vi "MoveScanFunc.vi"(6 "Multi ScanPar":bool[](array[boolean]), 7 "ActScanPar":bool[](array[boolean]), 8 "ErrorIn(No Error)":errorcluster caption="entrée d'erreur (pas d'erreur)", 9 "ScanFuncIn":string[][](array[string]), 10 "Dir(Up:T)":bool, 11 "Value":string) -> (0 "sortie d'erreur":errorcluster, 1 "ScanFuncOut":string[][](array[string]), 4 "Multi ScanParOut":bool[](array[boolean]), 5 "ActScanParOut":bool[](array[boolean]))   [LabVIEW 2019]
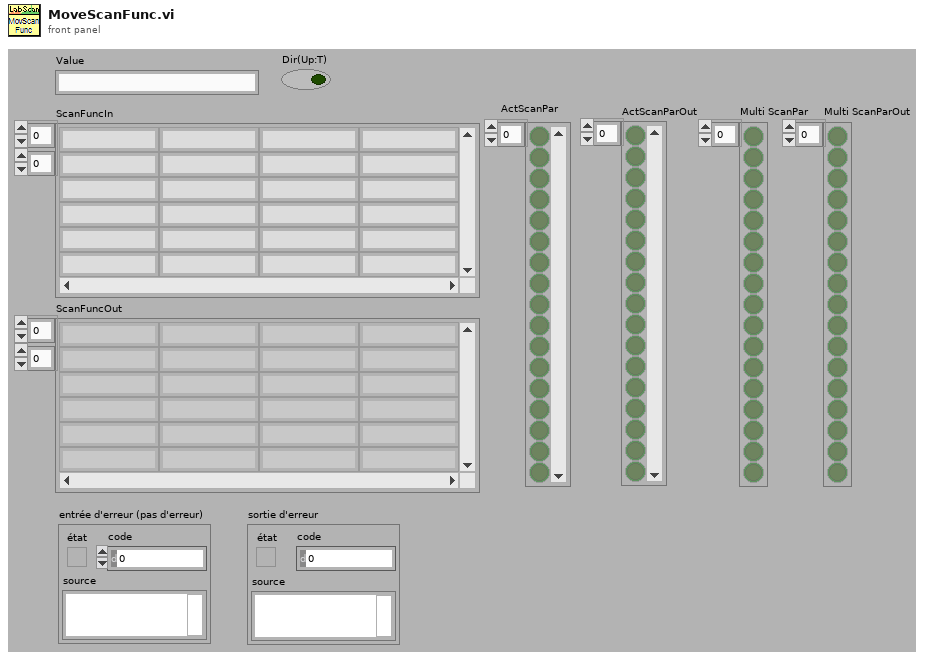
[diagram p1: front panel]
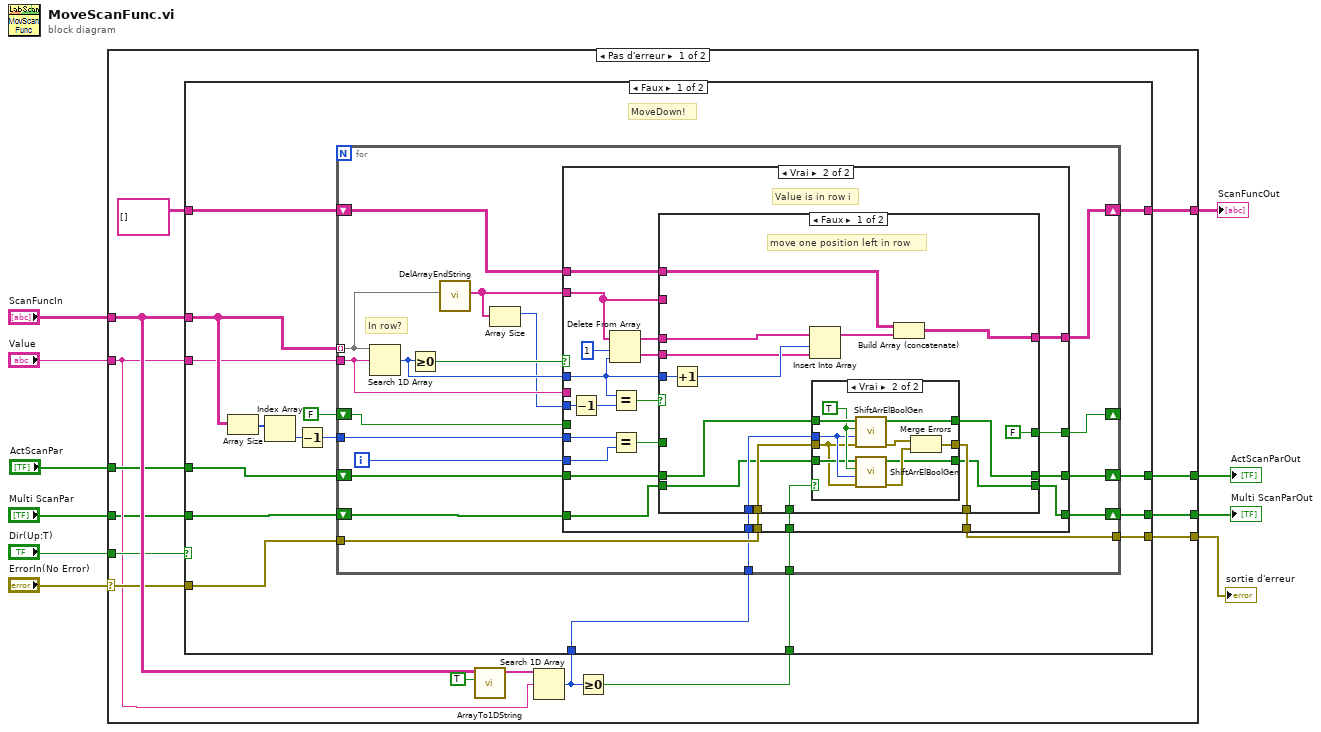
[diagram p0: block diagram]
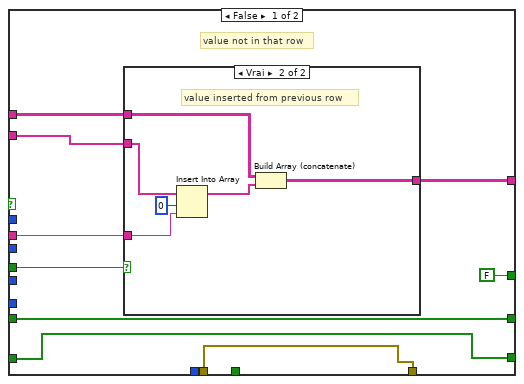
[diagram p2: hidden frame]
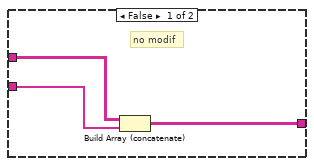
[diagram p3: hidden frame]
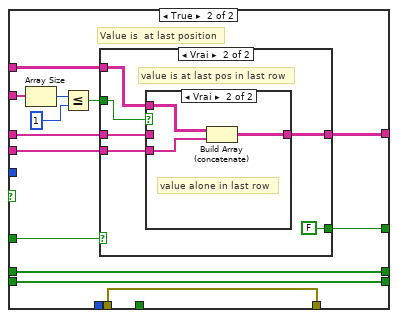
[diagram p5: hidden frame]
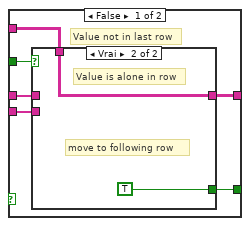
[diagram p6: hidden frame]
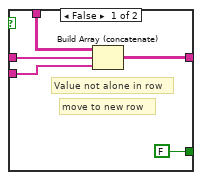
[diagram p7: hidden frame]
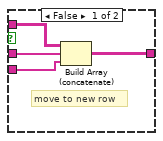
[diagram p8: hidden frame]
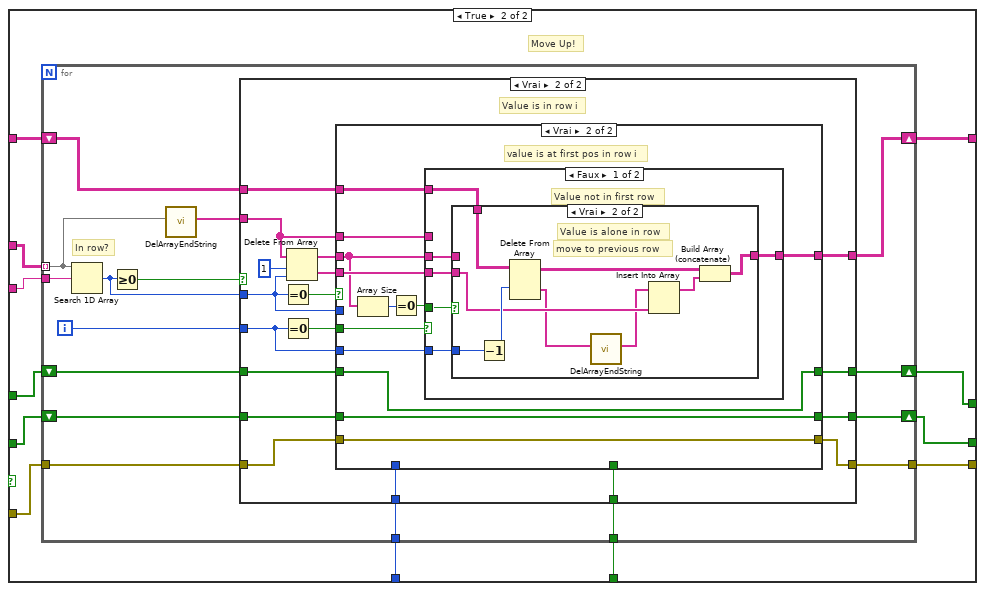
[diagram p9: hidden frame]
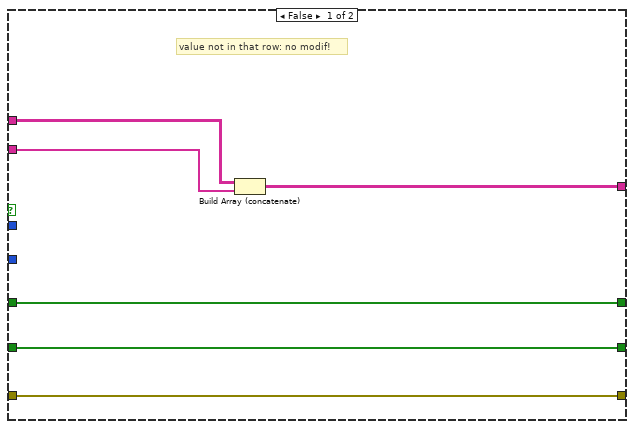
[diagram p10: hidden frame]
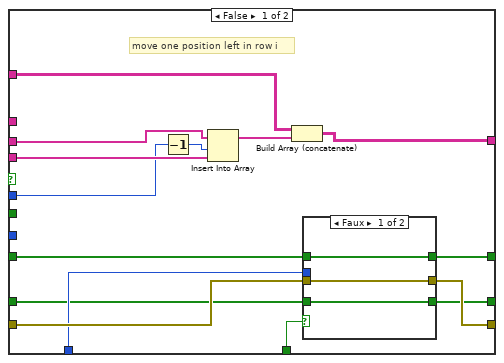
[diagram p11: hidden frame]
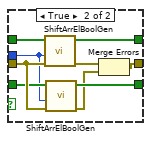
[diagram p12: hidden frame]
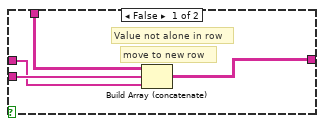
[diagram p13: hidden frame]
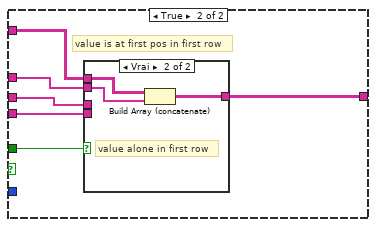
[diagram p14: hidden frame]
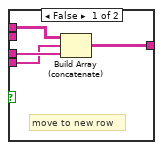
[diagram p15: hidden frame]
diagram:
  n1 = case shown="Pas d'erreur" "ErrorIn(No Error)" {
    selector: "ErrorIn(No Error)" -> [w20 w296]
    tunnel: "Value" -> [w13 _]
    tunnel: "ScanFuncIn" -> [w24 w295]
    tunnel: "Dir(Up:T)" -> [w21 _]
    tunnel: [w19 w296] -> w6
    tunnel: [w23 w295] -> w5
    tunnel: "ActScanPar" -> [w22 w294]
    tunnel: [w18 w294] -> w3
    tunnel: "Multi ScanPar" -> [w12 w293]
    tunnel: [w11 w293] -> w1
    frame No Error {
      n2 = call <userlib>:"ArrayTo1DString.vi"("DelArrEnd(F)"=TRUE ("DelArrEnd"), "tableau"=w24) -> ("Array Out"=w17:string[])  [unwired: 7 in, 2 out]
      n3 = Search 1D Array(1D array=w17, element=w13) -> (index of element=w14:i32)  [unwired: 1 in]
      n4 = Greater Or Equal To 0?(x=w14) -> (x >= 0?=w15:bool)
      n5 = case shown="Faux" w21 {
        tunnel: w13 -> [w31 w179]
        tunnel: string[][] [] -> [w41 w181]
        tunnel: [w40 w178] -> w23
        tunnel: w24 -> [w32 w180]
        tunnel: w22 -> [w28 w175]
        tunnel: w20 -> [w35 w176]
        tunnel: [w34 w177] -> w19
        tunnel: [w33 w173] -> w18
        tunnel: w15 -> [w30 w172]
        tunnel: w14 -> [w29 w174]
        tunnel: w12 -> [w27 w171]
        tunnel: [w26 w170] -> w11
        frame False {
          # "MoveDown!"
          n6 = Array Size(array=w32) -> (size(s)=w39:i32[])
          n7 = Index Array(array=w39) -> (element=w38:i32)  [unwired: 1 in]
          n8 = Decrement(x=w38) -> (x-1=w37:i32)
          n9 = for {
            tunnel: w32 -> [w52] mode=indexing
            tunnel: w31 -> [w53]
            shift-right: [w58] -> w40
            shift-left: w41 -> [w57]
            tunnel: w37 -> [w56]
            shift-right: [w55] -> _
            shift-left: FALSE -> [w54]
            tunnel: w35 -> [w49]
            tunnel: [w48] -> w34
            tunnel: w30 -> [w46]
            tunnel: w29 -> [w45]
            shift-right: [w47] -> w33
            shift-left: w28 -> [w44]
            shift-right: [w43] -> w26
            shift-left: w27 -> [w42]
            i -> [w59]
            # "In row?"
            n10 = Search 1D Array(1D array=w52, element=w53) -> (index of element=w60:i32)  [unwired: 1 in]
            n11 = Greater Or Equal To 0?(x=w60) -> (x >= 0?=w61:bool)
            n12 = call <userlib>:"DelArrayEndString.vi"("Array In"=w52) -> ("Array Out"=w50:string[])  [unwired: 9 in, 1 out]
            n13 = Array Size(array=w50) -> (size(s)=w51:i32)
            n14 = case shown="Vrai" w61 {
              tunnel: w60 -> [_ w88]
              tunnel: w50 -> [w68 w97]
              tunnel: [w69 w98] -> w58
              tunnel: w59 -> [_ w91]
              tunnel: w57 -> [w70 w96]
              tunnel: w51 -> [_ w95]
              tunnel: w56 -> [_ w92]
              tunnel: [FALSE w90] -> w55
              tunnel: w54 -> [w66 _]
              tunnel: w53 -> [w65 _]
              tunnel: w46 -> [_ w87]
              tunnel: w44 -> [w63 w82]
              tunnel: w49 -> [w64 w86]
              tunnel: w45 -> [_ w85]
              tunnel: [w64 w84] -> w48
              tunnel: [w63 w83] -> w47
              tunnel: [w62 w81] -> w43
              tunnel: w42 -> [w62 w80]
              frame False {
                # "value not in that row"
                n15 = case shown="Vrai" w66 {
                  tunnel: w70 -> [w73 w77]
                  tunnel: [w72 w75] -> w69
                  tunnel: w68 -> [w71 w79]
                  tunnel: w65 -> [_ w78]
                  frame False {
                    # "no modif"
                    n16 = Build Array (concatenate)(w73, w71) -> (w72:string[][])
                  }
                  frame True {
                    # "value inserted from previous row"
                    n17 = Insert Into Array(array=w79, index=0 ("indice"), new element=w78) -> (w76:string[])
                    n18 = Build Array (concatenate)(w77, w76) -> (w75:string[][])
                  }
                }
              }
              frame True {
                # "Value is in row i"
                n19 = Decrement(x=w95) -> (x-1=w89:i32)
                n20 = Delete From Array(array=w97, length=1 ("longueur"), index=w88) -> (deleted portion=w99:string[], array with subset deleted=w100:string[])
                n21 = Equal?(x=w88, y=w89) -> (x = y?=w94:bool)
                n22 = Equal?(x=w92, y=w91) -> (x = y?=w93:bool)
                n23 = case shown="Faux" w94 {
                  tunnel: w100 -> [w110 w139]
                  tunnel: w99 -> [w116 w142]
                  tunnel: w88 -> [w115 _]
                  tunnel: [w114 w141] -> w98
                  tunnel: w93 -> [_ w143]
                  tunnel: w97 -> [_ w137]
                  tunnel: w96 -> [w112 w140]
                  tunnel: [FALSE w134] -> w90
                  tunnel: w87 -> [w109 _]
                  tunnel: w82 -> [w104 w132]
                  tunnel: w86 -> [w108 w133]
                  tunnel: w85 -> [w107 _]
                  tunnel: [w106 w133] -> w84
                  tunnel: [w105 w132] -> w83
                  tunnel: [w102 w131] -> w81
                  tunnel: w80 -> [w103 w131]
                  frame False {
                    # "move one position left in row"
                    n24 = Increment(x=w115) -> (x+1=w117:i32)
                    n25 = Insert Into Array(array=w110, index=w117, new element=w116) -> (w113:string[])
                    n26 = case shown="Vrai" w109 {
                      tunnel: w104 -> [w120 w130]
                      tunnel: w108 -> [w119 w123]
                      tunnel: w107 -> [_ w127]
                      tunnel: [w119 w122] -> w106
                      tunnel: [w120 w129] -> w105
                      tunnel: w103 -> [w118 w124]
                      tunnel: [w118 w125] -> w102
                      frame False {
                      }
                      frame True {
                        w128 = TRUE ("Dir(DownFalse)")
                        n27 = call <userlib>:"ShiftArrElBoolGen.vi"("ErrorIn(No Error)"=w123, "Index"=w127, "Dir(DownFalse)"=w128, "Array In"=w130) -> ("sortie d'erreur"=w121:errorcluster, "Array Out"=w129:bool[])  [unwired: 5 in, 1 out]
                        n28 = call <userlib>:"ShiftArrElBoolGen.vi"("ErrorIn(No Error)"=w123, "Index"=w127, "Dir(DownFalse)"=w128, "Array In"=w124) -> ("sortie d'erreur"=w126:errorcluster, "Array Out"=w125:bool[])  [unwired: 5 in, 1 out]
                        n29 = Merge Errors(w121, w126) -> (w122:errorcluster)
                      }
                    }
                    n30 = Build Array (concatenate)(w112, w113) -> (w114:string[][])
                  }
                  frame True {
                    # "Value is  at last position"
                    n31 = Array Size(array=w137) -> (size(s)=w136:i32)
                    n32 = Less Or Equal?(x=w136, y=1) -> (x <= y?=w138:bool)
                    n33 = case shown="Vrai" w143 {
                      tunnel: w139 -> [w146 w158]
                      tunnel: w142 -> [w149 w159]
                      tunnel: [w148 w162] -> w141
                      tunnel: w140 -> [w147 w161]
                      tunnel: w138 -> [w145 w160]
                      tunnel: [w144 FALSE] -> w134
                      frame False {
                        # "Value not in last row"
                        n34 = case shown="Vrai" w145 {
                          tunnel: w149 -> [w152 _]
                          tunnel: [w154 w156] -> w148
                          tunnel: w147 -> [w153 w156]
                          tunnel: w146 -> [w151 _]
                          tunnel: [FALSE TRUE] -> w144
                          frame False {
                            # "Value not alone in row"
                            # "move to new row"
                            n35 = Build Array (concatenate)(w153, w151, w152) -> (w154:string[][])
                          }
                          frame True {
                            # "Value is alone in row"
                            # "move to following row"
                          }
                        }
                      }
                      frame True {
                        # "value is at last pos in last row"
                        n36 = case shown="Vrai" w160 {
                          tunnel: [w165 w169] -> w162
                          tunnel: w161 -> [w166 w168]
                          tunnel: w159 -> [w164 w167]
                          tunnel: w158 -> [w163 _]
                          frame False {
                            # "move to new row"
                            n37 = Build Array (concatenate)(w166, w163, w164) -> (w165:string[][])
                          }
                          frame True {
                            # "value alone in last row"
                            n38 = Build Array (concatenate)(w168, w167) -> (w169:string[][])
                          }
                        }
                      }
                    }
                  }
                }
              }
            }
          }
        }
        frame True {
          # "Move Up!"
          n39 = for {
            tunnel: w180 -> [w191] mode=indexing
            tunnel: w179 -> [w197]
            shift-right: [w193] -> w178
            shift-left: w181 -> [w192]
            tunnel: [w189] -> w177
            tunnel: w176 -> [w188]
            tunnel: w174 -> [w186]
            shift-right: [w185] -> w173
            shift-left: w175 -> [w187]
            tunnel: w172 -> [w184]
            shift-right: [w182] -> w170
            shift-left: w171 -> [w183]
            i -> [w194]
            # "In row?"
            n40 = Search 1D Array(1D array=w191, element=w197) -> (index of element=w195:i32)  [unwired: 1 in]
            n41 = Greater Or Equal To 0?(x=w195) -> (x >= 0?=w196:bool)
            n42 = call <userlib>:"DelArrayEndString.vi"("Array In"=w191) -> ("Array Out"=w190:string[])  [unwired: 9 in, 1 out]
            n43 = case shown="Vrai" w196 {
              tunnel: w195 -> [_ w217]
              tunnel: w190 -> [w201 w214]
              tunnel: [w202 w216] -> w193
              tunnel: w194 -> [_ w212]
              tunnel: w192 -> [w203 w213]
              tunnel: [w200 w210] -> w189
              tunnel: w188 -> [w200 w211]
              tunnel: [w199 w209] -> w185
              tunnel: w187 -> [w199 w208]
              tunnel: w186 -> [_ w207]
              tunnel: w184 -> [_ w206]
              tunnel: w183 -> [w198 w205]
              tunnel: [w198 w204] -> w182
              frame False {
                # "value not in that row: no modif!"
                n44 = Build Array (concatenate)(w203, w201) -> (w202:string[][])
              }
              frame True {
                # "Value is in row i"
                n45 = Equal To 0?(x=w217) -> (x = 0?=w220:bool)
                n46 = Equal To 0?(x=w212) -> (x = 0?=w215:bool)
                n47 = Delete From Array(array=w214, length=1 ("longueur"), index=w217) -> (deleted portion=w218:string[], array with subset deleted=w219:string[])
                n48 = case shown="Vrai" w220 {
                  tunnel: w219 -> [w233 w254]
                  tunnel: w218 -> [w235 w259]
                  tunnel: w217 -> [w234 _]
                  tunnel: [w232 w258] -> w216
                  tunnel: w215 -> [_ w260]
                  tunnel: w214 -> [_ w257]
                  tunnel: w213 -> [w230 w256]
                  tunnel: w212 -> [_ w255]
                  tunnel: w211 -> [w229 w251]
                  tunnel: [w228 w251] -> w210
                  tunnel: [w227 w250] -> w209
                  tunnel: w208 -> [w226 w250]
                  tunnel: w207 -> [w225 _]
                  tunnel: w206 -> [w224 _]
                  tunnel: w205 -> [w223 w249]
                  tunnel: [w222 w249] -> w204
                  frame False {
                    # "move one position left in row i"
                    n49 = Decrement(x=w234) -> (x-1=w236:i32)
                    n50 = Insert Into Array(array=w233, index=w236, new element=w235) -> (w231:string[])
                    n51 = Build Array (concatenate)(w230, w231) -> (w232:string[][])
                    n52 = case shown="Faux" w224 {
                      tunnel: w226 -> [w239 w248]
                      tunnel: w229 -> [w238 w245]
                      tunnel: w225 -> [_ w240]
                      tunnel: [w238 w243] -> w228
                      tunnel: [w239 w246] -> w227
                      tunnel: w223 -> [w237 w241]
                      tunnel: [w237 w244] -> w222
                      frame False {
                      }
                      frame True {
                        n53 = call <userlib>:"ShiftArrElBoolGen.vi"("ErrorIn(No Error)"=w245, "Index"=w240, "Array In"=w248) -> ("sortie d'erreur"=w247:errorcluster, "Array Out"=w246:bool[])  [unwired: 6 in, 1 out]
                        n54 = call <userlib>:"ShiftArrElBoolGen.vi"("ErrorIn(No Error)"=w245, "Index"=w240, "Array In"=w241) -> ("sortie d'erreur"=w242:errorcluster, "Array Out"=w244:bool[])  [unwired: 6 in, 1 out]
                        n55 = Merge Errors(w247, w242) -> (w243:errorcluster)
                      }
                    }
                  }
                  frame True {
                    # "value is at first pos in row i"
                    n56 = Array Size(array=w254) -> (size(s)=w253:i32)
                    n57 = Equal To 0?(x=w253) -> (x = 0?=w252:bool)
                    n58 = case shown="Faux" w260 {
                      tunnel: w254 -> [w263 w280]
                      tunnel: w259 -> [w266 w281]
                      tunnel: [w265 w285] -> w258
                      tunnel: w257 -> [_ w283]
                      tunnel: w256 -> [w264 w284]
                      tunnel: w255 -> [w262 _]
                      tunnel: w252 -> [w261 w282]
                      frame False {
                        # "Value not in first row"
                        n59 = case shown="Vrai" w261 {
                          tunnel: w266 -> [w270 w274]
                          tunnel: [w269 w271] -> w265
                          tunnel: w264 -> [w268 w278]
                          tunnel: w263 -> [w267 _]
                          tunnel: w262 -> [_ w279]
                          frame False {
                            # "Value not alone in row"
                            # "move to new row"
                            n60 = Build Array (concatenate)(w268, w270, w267) -> (w269:string[][])
                          }
                          frame True {
                            # "Value is alone in row"
                            # "move to previous row"
                            n61 = Decrement(x=w279) -> (x-1=w275:i32)
                            n62 = Delete From Array(array=w278, index (row)=w275) -> (deleted portion=w273:string[], array with subset deleted=w277:string[][])  [unwired: 2 in]
                            n63 = call <userlib>:"DelArrayEndString.vi"("Array In"=w273) -> ("Array Out"=w272:string[])  [unwired: 9 in, 1 out]
                            n64 = Insert Into Array(array=w272, new element=w274) -> (w276:string[])  [unwired: 1 in]
                            n65 = Build Array (concatenate)(w277, w276) -> (w271:string[][])
                          }
                        }
                      }
                      frame True {
                        # "value is at first pos in first row"
                        n66 = case shown="Vrai" w282 {
                          tunnel: [w288 w292] -> w285
                          tunnel: w284 -> [w289 w291]
                          tunnel: w283 -> [_ w290]
                          tunnel: w281 -> [w286 _]
                          tunnel: w280 -> [w287 _]
                          frame False {
                            # "move to new row"
                            n67 = Build Array (concatenate)(w289, w286, w287) -> (w288:string[][])
                          }
                          frame True {
                            # "value alone in first row"
                            n68 = Build Array (concatenate)(w291, w290) -> (w292:string[][])
                          }
                        }
                      }
                    }
                  }
                }
              }
            }
          }
        }
      }
    }
    frame Error {
    }
  }
  "sortie d'erreur" <- w6
  "ScanFuncOut" <- w5
  "ActScanParOut" <- w3
  "Multi ScanParOut" <- w1
